vi "Handle Notification.vi"(8 "error in":errorcluster, 9 "Payload":string, 10 "Notification Type":string, 11 "Plugin in":refnum<class "DFT_Spectra.lvclass">) -> (0 "error out":errorcluster, 3 "Plugin out":refnum<class "DFT_Spectra.lvclass">)   [LabVIEW 2024, in "DFT_Spectra.lvlib" / "DFT_Spectra.lvclass"]
uses:
  DFT_Spectra.lvclass
  DFT_Spectra.lvclass/DFT_Spectra.ctl
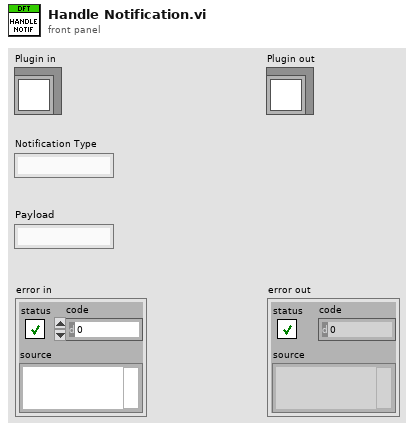
[diagram p1: front panel]
types:
  T1 = typedef "DFT_Spectra.lvlib/DFT_Spectra.lvclass/DFT_Spectra Data.ctl" = cluster{"First Time":bool, "Show Results Window":bool, "Show Results Window Clicked":bool, "Window":T2, "overlap":i32, "Block Duration":dbl, "Averaging parameters":cluster{"averaging mode":enum16{"No averaging", "Vector averaging", "RMS averaging", "Peak hold"}, "weighting mode":enum16{"Linear", "Exponential"}, "number of averages":u32}, "buffer out":refnum<data-value>, "Avg Spectra":refnum<vi>, "Spectra UI":refnum<vi>}
  T2 = typedef "NI_AALPro.lvlib/windowTd.ctl" = u32
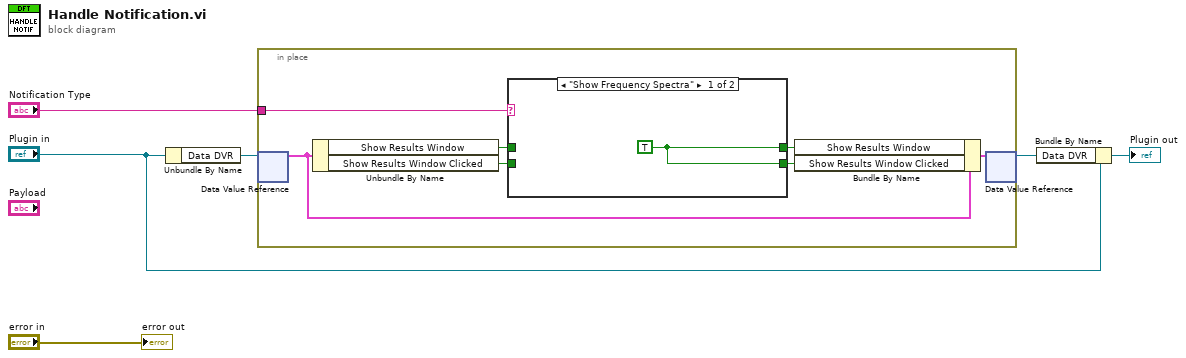
[diagram p0: block diagram]
diagram:
  n1 = Unbundle By Name("Plugin in") -> ("Data DVR"=w6:refnum<data-value>)
  n2 = in-place {
    in-place-border: "Notification Type" -> [w13]
    n3 = in-place-dvr #1(w6) -> (w10:T1)  [unwired: 1 out]
    n4 = Unbundle By Name(w10) -> ("Show Results Window"=w12:bool, "Show Results Window Clicked"=w11:bool)
    n5 = case shown="\"Show Frequency Spectra\"" w13 {
      tunnel: [w14 w16] -> w9
      tunnel: w12 -> [_ w16]
      tunnel: w11 -> [_ w15]
      tunnel: [w14 w15] -> w8
      frame "Show Frequency Spectra" {
        w14 = TRUE
      }
      frame Default {
      }
    }
    n6 = Bundle By Name(cluster=w10, "Show Results Window"=w9, "Show Results Window Clicked"=w8) -> (w7:T1)
    n7 = in-place-dvr #1(w7) -> (w5:refnum<data-value>)  [unwired: 1 out]
  }
  n8 = Bundle By Name(cluster="Plugin in", "Data DVR"=w5) -> (→"Plugin out":refnum<class "DFT_Spectra.lvclass">)
  "error out" <- "error in"
